vi "sub_Reconstruct Data Message.vi"(9 "Start Loc of Data":i32, 10 "Packet Info":T1, 11 "Input Stream":T2) -> (2 "Packet Info out":T1)   [LabVIEW 2011]
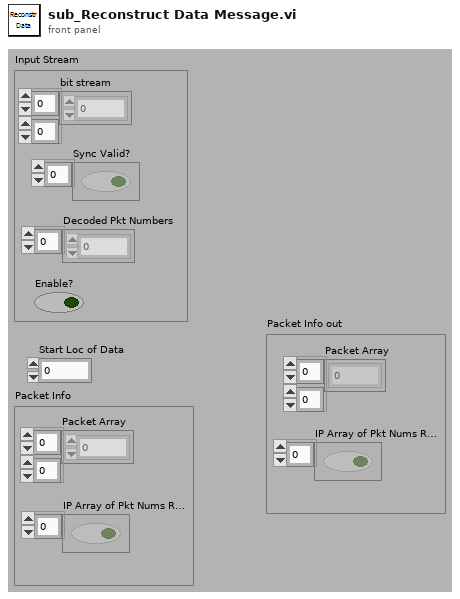
[diagram p1: front panel]
types:
  T1 = cluster{"Packet Array":i32[][], "IP Array of Pkt Nums Received  ":bool[]}
  T2 = cluster{"bit stream ":i8[][], "Sync Valid?":bool[], "Decoded Pkt Numbers":u32[], "Enable?":bool}
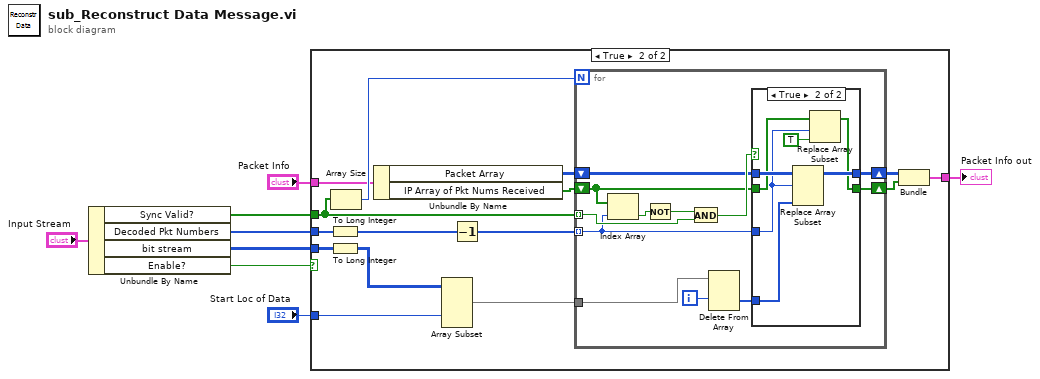
[diagram p0: block diagram]
diagram:
  n1 = Unbundle By Name("Input Stream") -> ("Sync Valid?"=w4:bool[], "Decoded Pkt Numbers"=w3:u32[], "bit stream"=w6:i8[][], "Enable?"=w5:bool)
  n2 = case shown="True" w5 {
    tunnel: w4 -> [_ w23]
    tunnel: w3 -> [_ w21]
    tunnel: w6 -> [_ w22]
    tunnel: "Start Loc of Data" -> [_ w18]
    tunnel: "Packet Info" -> [w9 w15]
    tunnel: [w9 w10] -> w1
    frame False {
    }
    frame True {
      n3 = To Long Integer(number=w21) -> (32bit integer=w20:i32[])
      n4 = To Long Integer(number=w22) -> (32bit integer=w17:i32[][])
      n5 = Array Size(array=w23) -> (size(s)=w24:i32)
      n6 = Unbundle By Name(w15) -> ("Packet Array"=w14:i32[][], "IP Array of Pkt Nums Received"=w13:bool[])
      n7 = Array Subset(array=w17, index (col)=w18) -> (w16:i32[][])  [unwired: 3 in]
      n8 = Decrement(x=w20) -> (x-1=w19:i32[])
      n9 = for {
        N: w24 -> [_]
        tunnel: w19 -> [w31] mode=indexing
        tunnel: w23 -> [w34] mode=indexing
        shift-right: [w29] -> w12
        shift-left: w14 -> [w28]
        shift-right: [w26] -> w11
        shift-left: w13 -> [w27]
        tunnel: w16 -> [w25]
        i -> [w33]
        n10 = Index Array(array=w27, index=w31) -> (element=w36:bool)
        n11 = Not(x=w36) -> (.not. x?=w35:bool)
        n12 = And(x=w35, y=w34) -> (x .and. y?=w32:bool)
        n13 = Delete From Array(array=w25, index (row)=w33) -> (deleted portion=w30:i32[])  [unwired: 2 in, 1 out]
        n14 = case shown="True" w32 {
          tunnel: w28 -> [w38 w45]
          tunnel: w31 -> [_ w41]
          tunnel: w30 -> [_ w44]
          tunnel: [w38 w43] -> w29
          tunnel: w27 -> [w37 w42]
          tunnel: [w37 w39] -> w26
          frame False {
          }
          frame True {
            n15 = Replace Array Subset(array=w45, new element=w44, index (row)=w41) -> (w43:i32[][])  [unwired: 1 in]
            n16 = Replace Array Subset(array=w42, new element=TRUE ("new element/subarray"), index=w41) -> (w39:bool[])
          }
        }
      }
      n17 = Bundle("Packet Array"=w12, "IP Array of Pkt Nums Received"=w11) -> (w10:T1)  [unwired: 1 in]
    }
  }
  "Packet Info out" <- w1
